vi "test.vi"() -> ()   [LabVIEW 2019, in "MD4Logger Engine.lvlib"]
uses:
  MD4Logger Engine.lvlib
panel:
  out "Error Out":errorcluster
  out "Error Out 2":errorcluster
  in  "Channels Count":i32=2
  in  "Path":path=path "C:/Users/Hovhannes/Desktop/MD4Logger/Source/Engine/DLL/WriterExample.dll"
  in  "MDF4 File Path":path=path "C:/Users/Hovhannes/Desktop/mfloggeddata/8x.mf4"
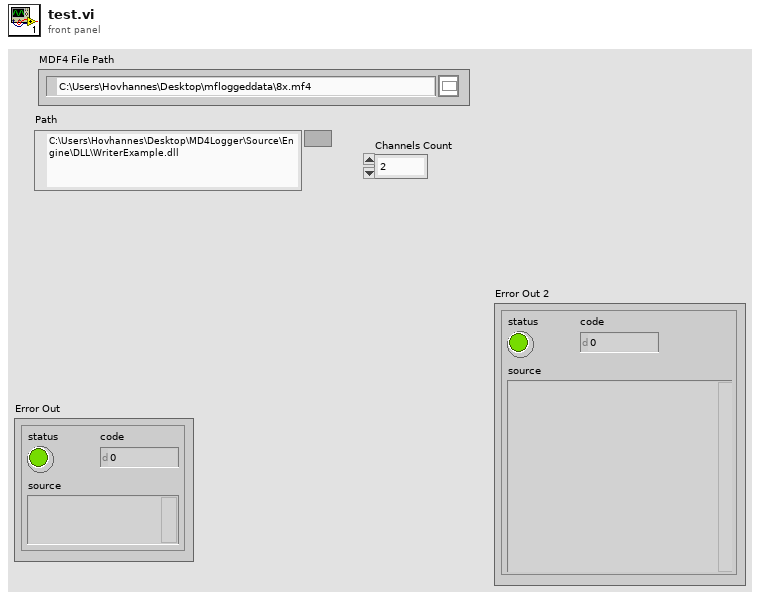
[diagram p1: front panel]
types:
  T1 = cluster{"Comment":string, "Time Source":string, "Author":string, "Department":string, "Project":string, "Subject":string}
  T2 = cluster{"History":string, "ID":string, "Vendor":string, "Version":string}
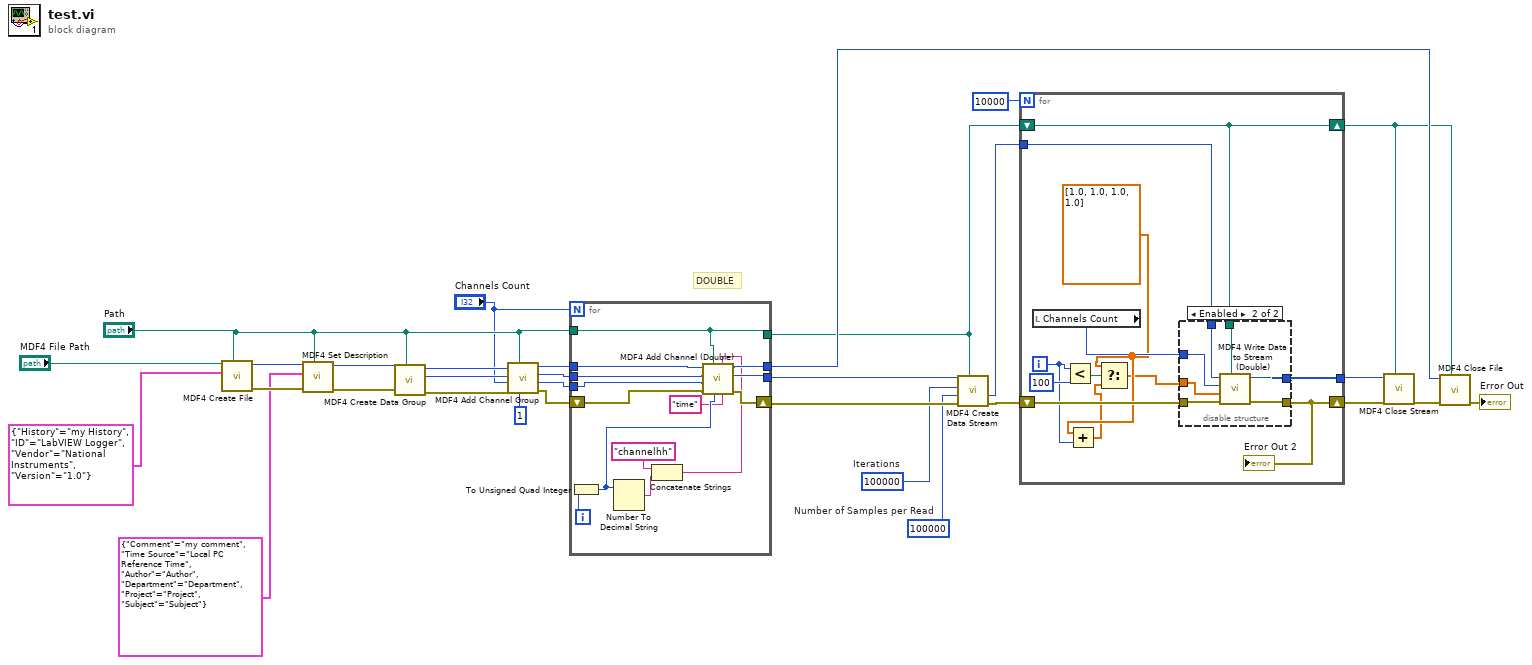
[diagram p0: block diagram]
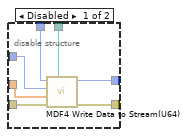
[diagram p2: hidden frame]
diagram:
  w6 = u32 100000  # Iterations
  w7 = u32 100000  # Number of Samples per Read
  # "DOUBLE"
  n1 = call "MDF4 Create File.vi"("path in"="Path", "History"=T2 {"History"="my History", "ID"="LabVIEW Logger", "Vendor"="National Instruments", "Version"="1.0"}, "MDF4 File Path"="MDF4 File Path") -> ("Error Out"=w29:errorcluster, "MDF4 File Reference out"=w30:i64)  [unwired: 6 in]
  n2 = call "MDF4 Set Description.vi"("path in"="Path", "Error In"=w29, "Comment"=T1 {"Comment"="my comment", "Time Source"="Local PC Reference Time", "Author"="Author", "Department"="Department", "Project"="Project", "Subject"="Subject"}, "MDF4 File Reference in"=w30) -> ("Error Out"=w28:errorcluster, "MDF4 File Reference out"=w27:i64)  [unwired: 6 in]
  n3 = call "MDF4 Create Data Group.vi"("path in"="Path", "Error In"=w28, "MDF4 File Reference in"=w27) -> ("Error Out"=w21:errorcluster, "Data Group Reference out"=w20:i64, "MDF4 File Reference out"=w19:i64)  [unwired: 6 in]
  n4 = call "MDF4 Add Channel Group.vi"("Record ID"=u64 1, "path in"="Path", "Error In"=w21, "chan_count"="Channels Count", "Data Group Reference in"=w20, "MDF4 File Reference in"=w19) -> ("Error Out"=w18:errorcluster, "Channel Group Reference out"=w16:i64, "Data Group Reference out"=w4:i64, "MDF4 File Reference out"=w17:i64)  [unwired: 2 in]
  n5 = for {
    N: "Channels Count" -> [_]
    tunnel: [w40] -> w22
    shift-right: [w41] -> w8
    shift-left: w18 -> [w42]
    tunnel: w17 -> [w36]
    tunnel: w4 -> [w35]
    tunnel: w16 -> [w34]
    tunnel: "Path" -> [w37]
    tunnel: [w37] -> w5
    tunnel: [w39] -> w3
    i -> [w43]
    n6 = To Unsigned Quad Integer(1:w43) -> (0:w33:u64)
    n7 = Number To Decimal String(number=w33) -> (decimal integer string=w45:string)  [unwired: 1 in]
    n8 = Concatenate Strings("channelhh" ("string"), w45) -> (w38:string)
    n9 = call "MDF4 Add Channel (Double).vi"("Channel Unit"="time", "Channel Name"=w38, "chan_index"=w33, "path in"=w37, "Error In"=w42, "Channel Group Reference in"=w34, "Data Group Reference in"=w35, "MDF4 File Reference in"=w36) -> ("Error Out"=w41:errorcluster, "Data Group Reference out"=w39:i64, "MDF4 File Reference out"=w40:i64)  [unwired: 1 in]
  }
  n10 = call "MDF4 Create Data Stream.vi"("path in"=w5, "Error In"=w8, "Number of Samples per Read"=w7, "Iterations"=w6, "Data Group Reference in"=w3) -> ("Error Out"=w10:errorcluster, "Stream Reference out"=w9:i64)  [unwired: 4 in, 1 out]
  n11 = for {
    N: 10000 -> [_]
    tunnel: w9 -> [w53]
    shift-right: [w57] -> w24
    shift-left: w10 -> [w55]
    shift-right: [w54] -> w13
    shift-left: w5 -> [w54]
    tunnel: [w56] -> w2
    i -> [w49]
    w48 = dbl[] [1.0, 1.0, 1.0, 1.0] ("data")
    n12 = local read "Channels Count"() -> (w52:i32)
    n13 = Less?(x=w49, y=100) -> (x < y?=w50:bool)
    n14 = Add(x=w48, y=w49) -> (x+y=w47:dbl[])
    n15 = Select(t=w48, s=w50, f=w47) -> (s? t:f=w46:dbl[])
    n16 = disable-structure shown="Enabled" {
      disable-tunnel: [w64 w70] -> w57
      disable-tunnel: [w63 w71] -> w56
      disable-tunnel: w55 -> [w62 w69]
      disable-tunnel: w54 -> [w61 w67]
      disable-tunnel: w53 -> [w60 w68]
      disable-tunnel: w52 -> [w59 w66]
      disable-tunnel: w46 -> [w58 w65]
      frame Disabled {
        n17 = call "MDF4 Write Data to Stream(U64).vi"("path in"=w61, "Error In"=w62, "data"=w58, "chan_count"=w59, "Stream Reference in"=w60) -> ("Error Out"=w64:errorcluster, "Stream Reference out"=w63:i64)  [unwired: 5 in]
      }
      frame Enabled {
        n18 = call "MDF4 Write Data to Stream (Double).vi"("path in"=w67, "Error In"=w69, "data"=w65, "chan_count"=w66, "Stream Reference in"=w68) -> ("Error Out"=w70:errorcluster, "Stream Reference out"=w71:i64)  [unwired: 5 in]
      }
    }
    "Error Out 2" <- w57
  }
  n19 = call "MDF4 Close Stream.vi"("path in"=w13, "Error In"=w24, "Stream Reference in"=w2) -> ("Error Out"=w23:errorcluster)  [unwired: 7 in, 1 out]
  n20 = call "MDF4 Close File.vi"("path in"=w13, "Error In"=w23, "MDF4 File Reference in"=w22) -> ("Error Out"=→"Error Out":errorcluster)  [unwired: 7 in, 1 out]
